vi "Load Config.vi"(8 "error in (no error)":errorcluster, 11 "Motion Controller in":refnum<class "Parent SIM Motion Controller.lvclass">) -> (0 "error out":errorcluster, 3 "Motion Controller out":refnum<class "Parent SIM Motion Controller.lvclass">)   [LabVIEW 2022 SP3, in "Parent SIM Motion Controller.lvclass"]
uses:
  Parent SIM Motion Controller.lvclass
  C:/Stage-Work/MAS/Framework/Base/Base.lvclass
  Framework/Base/Base.lvclass/Base.ctl
  Parent SIM Motion Controller.lvclass/Parent SIM Motion Controller.ctl
  0eb4f123-3beb-4f63-9979-2ce17083ca5a.vi
  Framework/Base/Accessors/Read Config Path.vi
  Framework/Base/Accessors/Read Section.vi
  <vilib>/Utility/config.llb/Open Config Data.vi
  <userlib>/_OpenG.lib/variantconfig/variantconfig.llb/Read Section Cluster__ogtk.vi
  <vilib>/Utility/config.llb/Close Config Data.vi
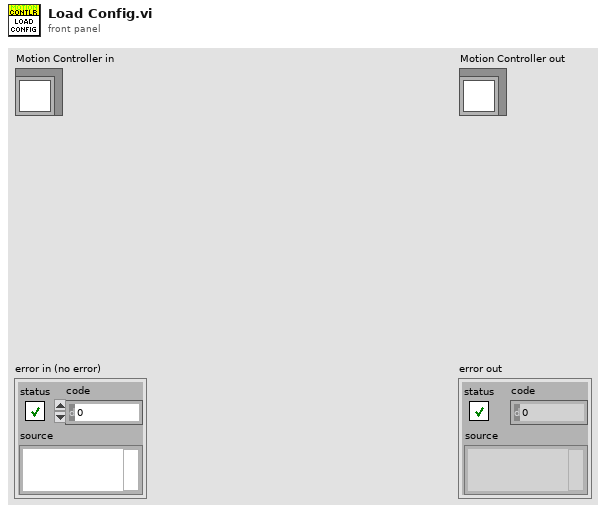
[diagram p1: front panel]
types:
  T1 = typedef "Parent SIM Motion Controller.lvclass/Settings.ctl" = cluster{"Axis Name":string}
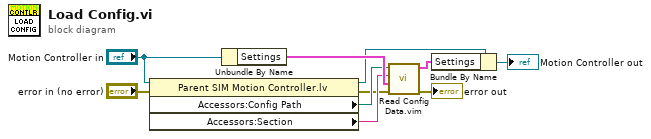
[diagram p0: block diagram]
diagram:
  n1 = property class="Parent SIM Motion Controller.lv"(reference="Motion Controller in", error in="error in (no error)") -> (reference out=w8:refnum<class "Parent SIM Motion Controller.lvclass">, error out=w1:errorcluster, "Accessors:Config Path"=w7:path, "Accessors:Section"=w6:string)
  n2 = Unbundle By Name("Motion Controller in") -> ("Settings"=w9:T1)
  n3 = call "Read Config Data.vim"("error in (no error)"=w1, "Section Formatted Cluster Type"=w9, "Section"=w6, "Config Path"=w7) -> ("error out"=→"error out":errorcluster, "Section Formatted Cluster Type 2"=w4:T1)  [unwired: 6 in]
  n4 = Bundle By Name(cluster=w8, "Settings"=w4) -> (→"Motion Controller out":refnum<class "Parent SIM Motion Controller.lvclass">)
